vi "RobotArm_Communication.vi"() -> ()   [LabVIEW 2018]
panel:
  out "Numeric 2":i32
  out "Numeric":i32
  out "data out":string
  out "error out 2":errorcluster
  in  "Send":bool
  in  "data in":string
  in  "stop 2":bool
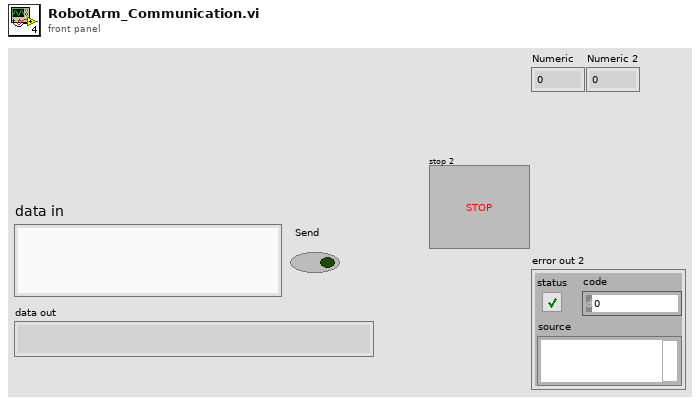
[diagram p1: front panel]
types:
  T1 = enum16{"Standard", "Buffered", "CRLF", "Immediate"}
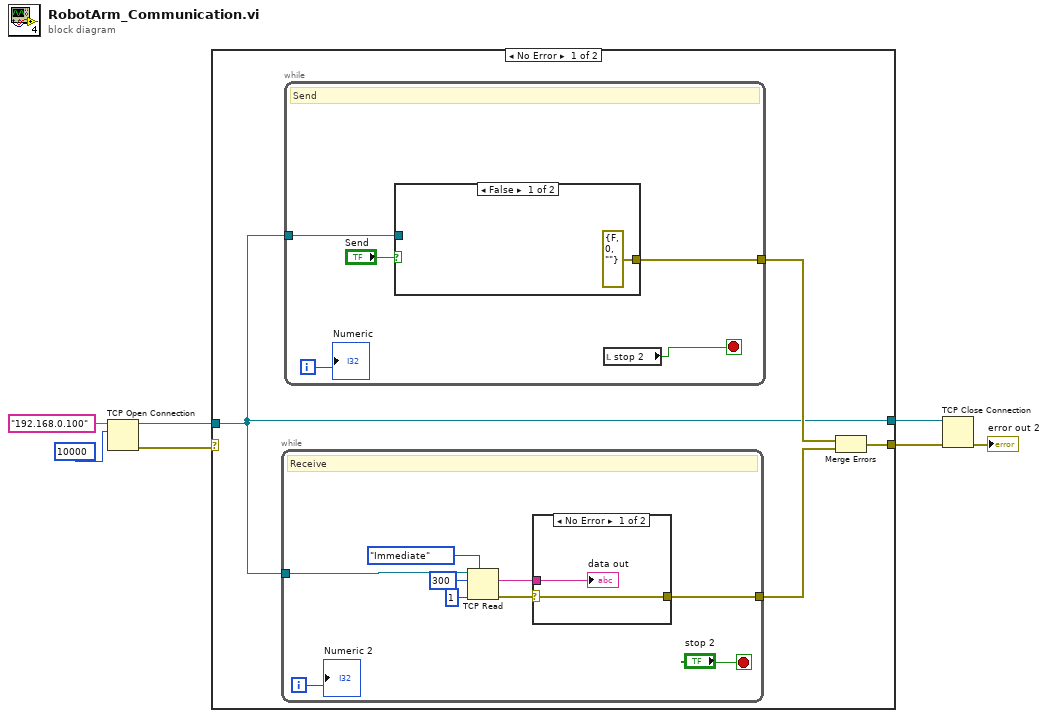
[diagram p0: block diagram]
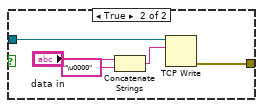
[diagram p3: hidden frame]
diagram:
  n1 = TCP Open Connection(address="192.168.0.100", remote port or service name=u16 10000) -> (connection ID=w5:refnum<k5>, error out=w4:errorcluster)  [unwired: 3 in]
  n2 = case shown="No Error" w4 {
    selector: w4 -> [_ w35]
    tunnel: w5 -> [w8 w36]
    tunnel: [w9 w35] -> w2
    tunnel: [w8 w36] -> w1
    frame No Error {
      n3 = while {
        tunnel: w8 -> [w17]
        tunnel: [w14] -> w11
        i -> [w15]
        stop <- "stop 2" stop-if-true
        # "Receive"
        n4 = TCP Read(connection ID=w17, bytes to read=300, 7:T1."Immediate" ("mode (standard)"), 9:1 ("timeout ms (25000)")) -> (data out=w20:string, error out=w16:errorcluster)  [unwired: 1 in, 1 out]
        n5 = case shown="No Error" w16 {
          selector: w16 -> [w21 w23]
          tunnel: w20 -> [w22 _]
          tunnel: [w21 w23] -> w14
          frame No Error {
            "data out" <- w22
          }
          frame Error {
          }
        }
        "Numeric 2" <- w15
      }
      n6 = while {
        tunnel: w8 -> [w28]
        tunnel: [w25] -> w10
        i -> [w27]
        stop <- w24 stop-if-true
        # "Send"
        n7 = case shown="False" "Send" {
          tunnel: w28 -> [_ w34]
          tunnel: [errorcluster {"status"=FALSE, "code"=0, "source"=""} ("error out") w33] -> w25
          frame False {
          }
          frame True {
            n8 = Concatenate Strings("data in", "\u0000" ("string")) -> (w30:string)
            n9 = TCP Write(connection ID=w34, data in=w30) -> (error out=w33:errorcluster)  [unwired: 2 in, 2 out]
          }
        }
        n10 = local read "stop 2"() -> (w24:bool)
        "Numeric" <- w27
      }
      n11 = Merge Errors(w10, w11) -> (w9:errorcluster)
    }
    frame Error {
    }
  }
  n12 = TCP Close Connection(connection ID=w1, error in (no error)=w2) -> (error out=→"error out 2":errorcluster)  [unwired: 1 in, 1 out]
